vi "Check Status (No Objects).vi"(8 "error in (no error)":errorcluster, 11 "Cluster In":T1) -> (0 "error out":errorcluster, 1 "Status":string, 2 "Ready?":bool, 3 "Cluster Out":T1)   [LabVIEW 2009]
doc: "Checks if the instrument is powered on and updates its member data with the instrument's current status."
uses:
  LCD Retarder.lvclass
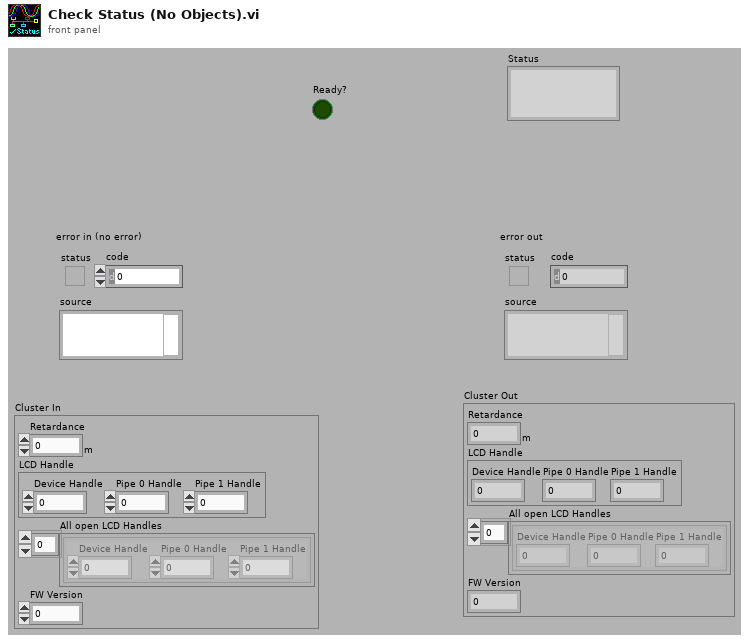
[diagram p1: front panel]
types:
  T1 = cluster{"Retardance":dbl[unit], "LCD Handle":cluster{"Device Handle":u32, "Pipe 0 Handle":u32, "Pipe 1 Handle":u32}, "All open LCD Handles":cluster{"Device Handle":u32, "Pipe 0 Handle":u32, "Pipe 1 Handle":u32}[], "FW Version":dbl}
  T2 = typedef "Readable.lvclass/X array.ctl" = T3[]
  T3 = typedef "Readable.lvclass/X.ctl" = dbl
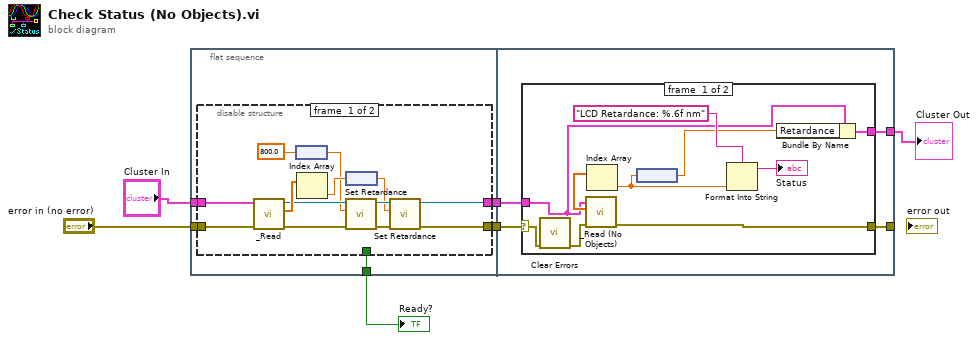
[diagram p0: block diagram]
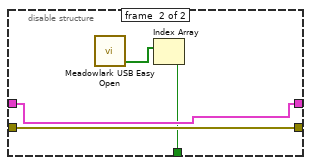
[diagram p2: hidden frame]
diagram:
  n1 = flat-sequence {
    tunnel: "error in (no error)" -> [w10]
    tunnel: "Cluster In" -> [w11]
    tunnel: [w9] -> w6
    tunnel: [w8] -> w5
    tunnel: [w7] -> w4
    tunnel: [w32] -> w1
    tunnel: [w30] -> _
    tunnel: w6 -> [w31]
    tunnel: w5 -> [w29]
    frame #0 {
      n2 = disable-structure shown="Enabled" {
        disable-tunnel: w11 -> [w23 w27]
        disable-tunnel: w10 -> [w22 w26]
        disable-tunnel: [w16 w27] -> w9
        disable-tunnel: [w12 w26] -> w8
        disable-tunnel: [_ w25] -> w7
        frame #0 {
          n3 = call-dynamic "_Read.vi"("errorIN"=w22, "LCD in"=w23) -> ("errorOUT"=w18:errorcluster, "X array"=w21:T2, "LCD out"=w15:refnum<class "LCD Retarder.lvclass">)  [unwired: 7 out]
          n4 = node(800.0) -> (w13:dbl[unit])
          n5 = Index Array(array=w21) -> (element=w20:T3)  [unwired: 1 in]
          n6 = node(w20) -> (w19:dbl[unit])
          n7 = call "Set Retardance.vi"("errorIN"=w18, "Retardance"=w13, "LCD in"=w15) -> ("errorOUT"=w17:errorcluster, "LCD out"=w24:refnum<class "LCD Retarder.lvclass">)  [unwired: 6 in, 1 out]
          n8 = call "Set Retardance.vi"("errorIN"=w17, "Retardance"=w19, "LCD in"=w24) -> ("errorOUT"=w12:errorcluster, "LCD out"=w16:refnum<class "LCD Retarder.lvclass">)  [unwired: 6 in, 1 out]
        }
        frame #1 {
          n9 = call "Meadowlark USB Easy Open.vi"() -> ("Device Opened Array"=w28:bool[])  [unwired: 2 out]
          n10 = Index Array(array=w28) -> (element=w25:bool)  [unwired: 1 in]
        }
      }
    }
    frame #1 {
      n11 = case shown="No Error" w29 {
        selector: w29 -> [w35 w43]
        tunnel: [w42 w43] -> w30
        tunnel: w31 -> [w33 w44]
        tunnel: [w39 w44] -> w32
        frame #0 {
          n12 = call <vilib>:"Clear Errors.vi"("error in (no error)"=w35) -> ("error out"=w34:errorcluster)  [unwired: 6 in]
          n13 = call "_Read (No Objects).vi"("errorIN"=w34, "Cluster In"=w33) -> ("errorOUT"=w42:errorcluster, "X array"=w38:T2)  [unwired: 7 in, 1 out]
          n14 = Index Array(array=w38) -> (element=w36:T3)  [unwired: 1 in]
          n15 = node(w36) -> (w37:dbl[unit])
          n16 = Format Into String(format string="LCD Retardance: %.6f nm", w36) -> (resulting string=→"Status":string)  [unwired: 2 in, 1 out]
          n17 = Bundle By Name(cluster=w33, "Retardance"=w37) -> (w39:T1)
        }
        frame #1 {
        }
      }
    }
  }
  "Ready?" <- w4
  "Cluster Out" <- w1
